vi "EX 5-2 Light Show.vi"() -> ()   [LabVIEW 2011, in "LabVIEW Interface for Arduino.lvlib"]
doc: "An Example that uses an Arduino to control Tri Colored LEDs (or BlinkM's) based on wav audio data."
uses:
  <vilib>/LabVIEW Interface for Arduino/LabVIEW Interface for Arduino.lvlib
panel:
  out "Levels":dbl[](graph)
  out "Raw Sound Data":waveform(dbl)[](graph)
  in  "Cycle Colors":bool
  in  "Stop":bool
  in  "Samples Per Read":i32=3000
  in  "Start Position":i32
  in  ".wav File":path
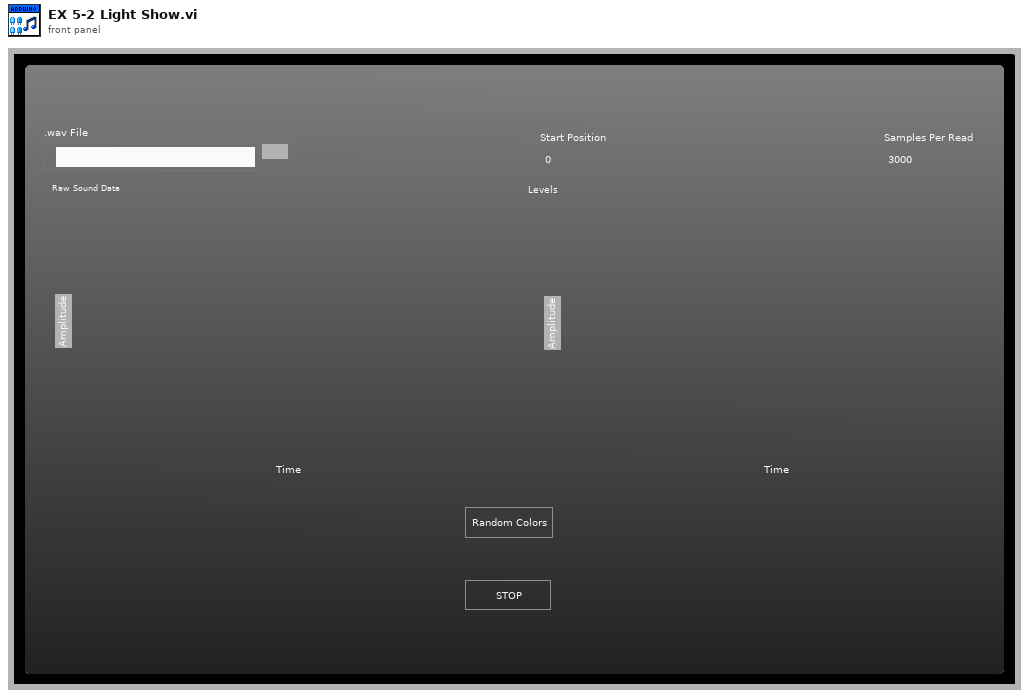
[diagram p1: front panel]
types:
  T1 = typedef "LabVIEW Interface for Arduino.lvlib/Arduino Resource.ctl" = cluster{"VISA resource":refnum<visa-resource-name>, "Board Type":T2, "Connection Type":enum8{"USB / Serial"}, "Bytes Per Packet (15)":u8}
  T2 = typedef "LabVIEW Interface for Arduino.lvlib/Board Type.ctl" = enum16{"Uno", "Dimuelanove w/Atmega 328", "Mega 2560"}
  T3 = typedef "Sound Output Task ID.ctl" = u32
  T4 = typedef "Sound File Refnum.ctl" = refnum<file>
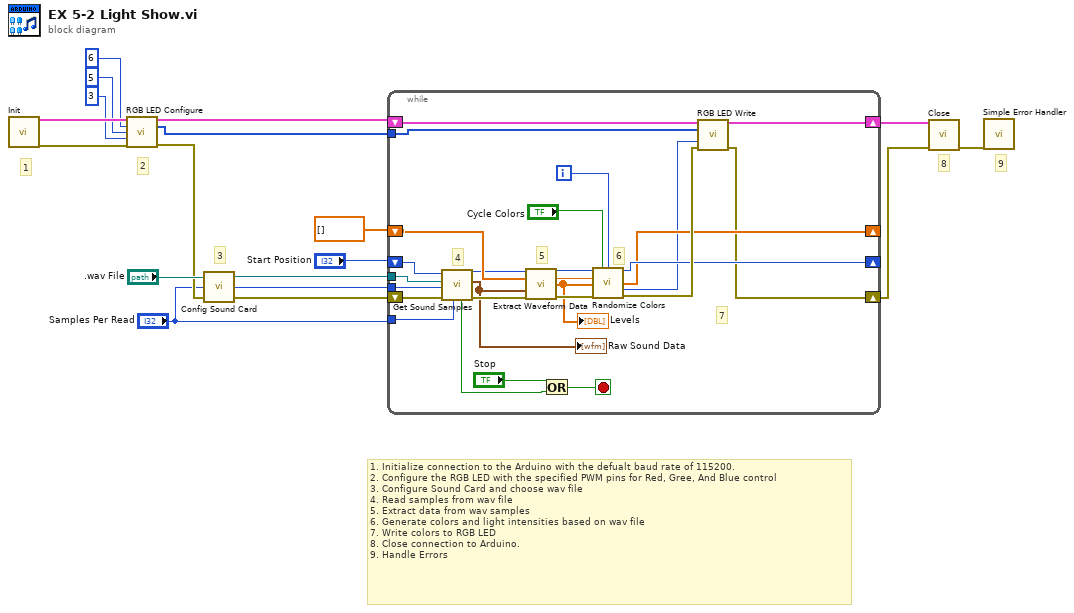
[diagram p0: block diagram]
diagram:
  # "9"
  # "8"
  # "3"
  # "2"
  # "1"
  # "1. Initialize connection to the Arduino with the defualt baud rate of 115200.\n2. Configure the RGB LED with the specified PWM pins for Red, Gree, And Blue control\n3. Configure Sound Card and choose wav file\n4. Read samples from wav file\n5. Extract data from wav samples\n6. Generate colors and light intensities based on wav file\n7. Write colors to RGB LED\n8. Close connection to Arduino.\n9. Handle Errors"
  n1 = call <vilib>:"Init.vi"() -> ("Arduino Resource"=w7:T1, "error out"=w6:errorcluster)  [unwired: 18 in]
  n2 = call <vilib>:"RGB LED Configure.vi"("Arduino Resource"=w7, "Red Pin"=6, "Green Pin"=5, "Blue Pin"=3, "error in"=w6) -> ("Arduino Resource"=w14:T1, "RGB LED Pins"=w1:u8[], "error out"=w11:errorcluster)  [unwired: 8 in]
  n3 = call <vilib>:"Config Sound Card.vi"("error in"=w11, "Samples Per Read"="Samples Per Read", "Song"=".wav File") -> ("error out"=w15:errorcluster, "task ID"=w18:T3, "sound file refnum"=w17:T4)
  n4 = while {
    shift-right: [w22] -> w13
    shift-left: w15 -> [w44]
    shift-right: [w34] -> _
    shift-left: "Start Position" -> [w40]
    shift-right: [w33] -> _
    shift-left: dbl[] [] -> [w31]
    shift-right: [w21] -> w5
    shift-left: w14 -> [w20]
    tunnel: "Samples Per Read" -> [w38]
    tunnel: w17 -> [w41]
    tunnel: w18 -> [w42]
    tunnel: w1 -> [w19]
    i -> [w43]
    stop <- w28 stop-if-true
    # "7"
    # "6"
    # "5"
    # "4"
    n5 = call <vilib>:"Get Sound Samples.vi"("error in"=w44, "task ID"=w42, "sound file refnum"=w41, "Sample Start Position"=w40, "Samples Per Read"=w38) -> ("end of file?"=w39:bool, "error out"=w37:errorcluster, "data"=w24:waveform(dbl)[], "Next Sample Start Position"=w29:i32)  [unwired: 2 in]
    "Raw Sound Data" <- w24
    n6 = call <vilib>:"Extract Waveform Data.vi"("Next Sample Start Position"=w29, "Previous Amplitudes"=w31, "data"=w24, "error in"=w37) -> ("Next Sample Start Position"=w30:i32, "Current Max"=w32:dbl, "Levels"=w23:dbl[], "error out"=w36:errorcluster)  [unwired: 8 in]
    "Levels" <- w23
    n7 = Or(x="Stop", y=w39) -> (x .or. y?=w28:bool)
    n8 = call <vilib>:"Randomize Colors.vi"("Next Sample Start Position"=w30, "Cycle Colors?"="Cycle Colors", "Iteration"=w43, "Current Max"=w32, "Levels"=w23, "error in"=w36) -> ("Next Sample Start Position"=w34:i32, "Levels"=w33:dbl[], "Color"=w27:u32, "error out"=w35:errorcluster)  [unwired: 6 in]
    n9 = call <vilib>:"RGB LED Write.vi"("Arduino Resource"=w20, "RGB LED Pins"=w19, "Color"=w27, "error in"=w35) -> ("Arduino Resource"=w21:T1, "error out"=w22:errorcluster)  [unwired: 9 in, 1 out]
  }
  n10 = call <vilib>:"Close.vi"("Arduino Resource"=w5, "error in"=w13) -> ("error out"=w12:errorcluster)  [unwired: 13 in]
  n11 = call <vilib>:"Simple Error Handler.vi"("error in (no error)"=w12) -> ()  [unwired: 4 in, 5 out]
